vi "Reclosing_R2.vi"(5 "Recloser Settings":T1, 6 "Counter In":dbl, 7 "y":dbl, 8 "Reclose In":bool, 9 "RMS values":dbl[](array[numeric]), 10 "PLL output":cluster{dbl, dbl, dbl, dbl}, 11 "Reclose?":bool) -> (0 "Phase difference":dbl, 1 "frequency difference":dbl, 2 "magnitude difference":dbl, 3 "Recloser action":bool, 4 "Counter Out":dbl)   [LabVIEW 2016]
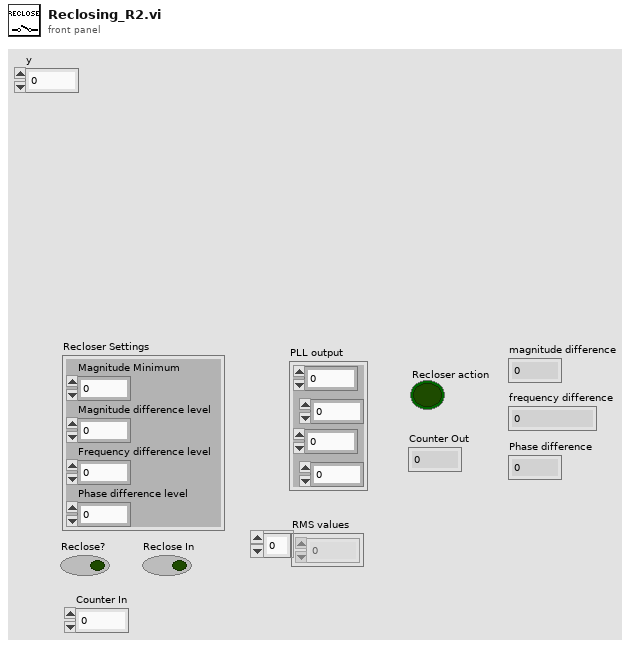
[diagram p1: front panel]
types:
  T1 = cluster{"Magnitude Minimum":dbl, "Magnitude difference level":dbl, "Frequency difference level":dbl, "Phase difference level":dbl}
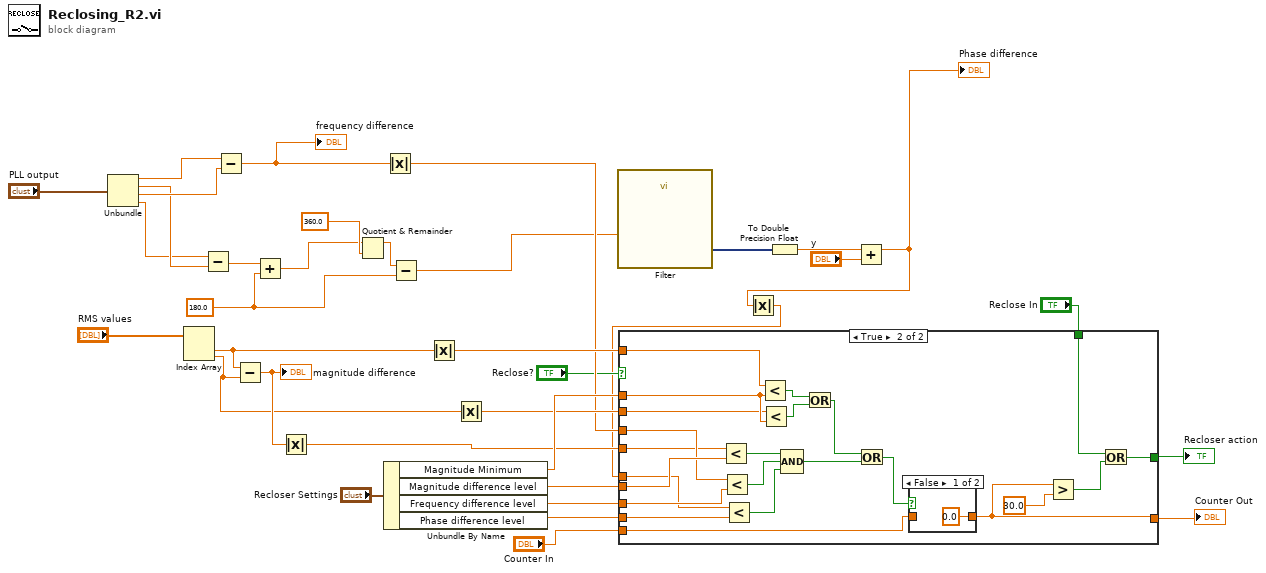
[diagram p0: block diagram]
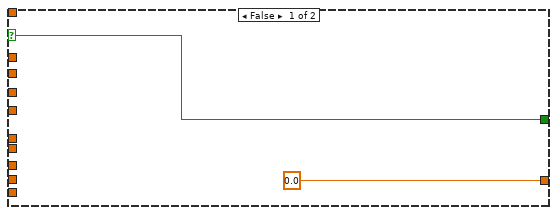
[diagram p2: hidden frame]
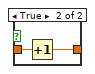
[diagram p3: hidden frame]
diagram:
  w29 = 180.0 ("y")
  n1 = Unbundle("PLL output") -> (w19:dbl, w17:dbl, w18:dbl, w16:dbl)
  n2 = Index Array(array="RMS values") -> (element #1=w13:dbl, element #2=w12:dbl)  [unwired: 2 in]
  n3 = Subtract(x=w16, y=w17) -> (x-y=w35:dbl)
  n4 = Subtract(x=w19, y=w18) -> (x-y=w15:dbl)
  "frequency difference" <- w15
  n5 = Subtract(x=w13, y=w12) -> (x-y=w24:dbl)
  "magnitude difference" <- w24
  n6 = Add(x=w35, y=w29) -> (x+y=w31:dbl)
  n7 = Absolute Value(x=w24) -> (abs(x)=w7:dbl)
  n8 = Quotient & Remainder(x=w31, y=360.0) -> (x-y*floor(x/y)=w33:dbl)  [unwired: 1 out]
  n9 = Unbundle By Name("Recloser Settings") -> ("Magnitude Minimum"=w28:dbl, "Magnitude difference level"=w27:dbl, "Frequency difference level"=w26:dbl, "Phase difference level"=w25:dbl)
  n10 = Absolute Value(x=w15) -> (abs(x)=w21:dbl)
  n11 = Subtract(x=w33, y=w29) -> (x-y=w4:dbl)
  n12 = Absolute Value(x=w13) -> (abs(x)=w22:dbl)
  n13 = Absolute Value(x=w12) -> (abs(x)=w23:dbl)
  n14 = call "Filter"("Signal"=w4) -> ("Filtered Signal"=w32:dynamicdata)  [unwired: 9 in, 1 out]
  n15 = To Double Precision Float(number=w32) -> (double precision float=w5:dbl)
  n16 = Add(x=w5, y="y") -> (x+y=w1:dbl)
  "Phase difference" <- w1
  n17 = Absolute Value(x=w1) -> (abs(x)=w2:dbl)
  n18 = case shown="True" "Reclose?" {
    selector: "Reclose?" -> [w37 _]
    tunnel: [w37 w38] -> w8
    tunnel: [0.0 w42] -> w9
    tunnel: w28 -> [_ w53]
    tunnel: w27 -> [_ w52]
    tunnel: w26 -> [_ w51]
    tunnel: w25 -> [_ w50]
    tunnel: w2 -> [_ w49]
    tunnel: w21 -> [_ w48]
    tunnel: w7 -> [_ w47]
    tunnel: "Counter In" -> [_ w46]
    tunnel: w22 -> [_ w45]
    tunnel: w23 -> [_ w44]
    tunnel: "Reclose In" -> [_ w40]
    frame False {
    }
    frame True {
      n19 = Less?(x=w47, y=w52) -> (x < y?=w55:bool)
      n20 = Less?(x=w48, y=w51) -> (x < y?=w58:bool)
      n21 = Less?(x=w49, y=w50) -> (x < y?=w57:bool)
      n22 = Less?(x=w45, y=w53) -> (x < y?=w60:bool)
      n23 = Less?(x=w44, y=w53) -> (x < y?=w59:bool)
      n24 = Compound Arithmetic op=AND(w55, w58, w57) -> (w56:bool)
      n25 = Or(x=w60, y=w59) -> (x .or. y?=w54:bool)
      n26 = Or(x=w54, y=w56) -> (x .or. y?=w41:bool)
      n27 = case shown="False" w41 {
        tunnel: [0.0 w63] -> w42
        tunnel: w46 -> [_ w62]
        frame False {
        }
        frame True {
          n28 = Increment(x=w62) -> (x+1=w63:dbl)
        }
      }
      n29 = Greater?(x=w42, y=30.0 ("x")) -> (0:w39:bool)
      n30 = Or(x=w40, y=w39) -> (x .or. y?=w38:bool)
    }
  }
  "Recloser action" <- w8
  "Counter Out" <- w9
